vi "Write Heading Data to TDMS.vi"(8 "error in (no error)":errorcluster, 10 "Heading Data":T1, 11 "Honeywell Compass HMC6343":refnum<class "Honeywell Compass HMC6343.lvclass">) -> (0 "error out":errorcluster, 3 "Honeywell Compass HMC6343 out":refnum<class "Honeywell Compass HMC6343.lvclass">)   [LabVIEW 2019, in "Honeywell Compass HMC6343.lvclass"]
doc: "Writes Heading Data to TDMS file."
uses:
  Honeywell Compass HMC6343.lvclass
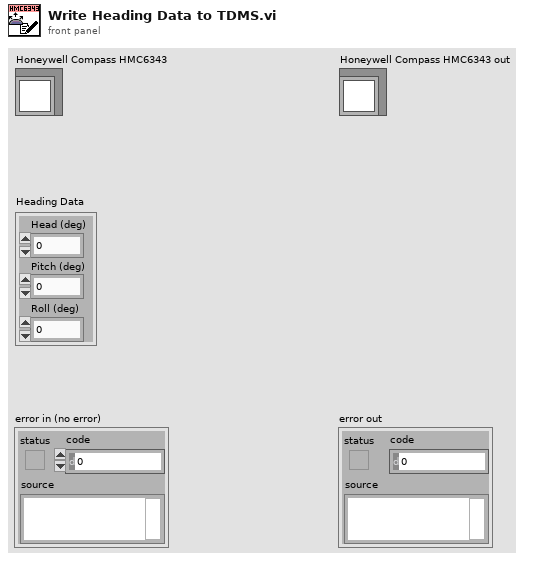
[diagram p1: front panel]
types:
  T1 = cluster{"Head (deg)":dbl, "Pitch (deg)":dbl, "Roll (deg)":dbl}
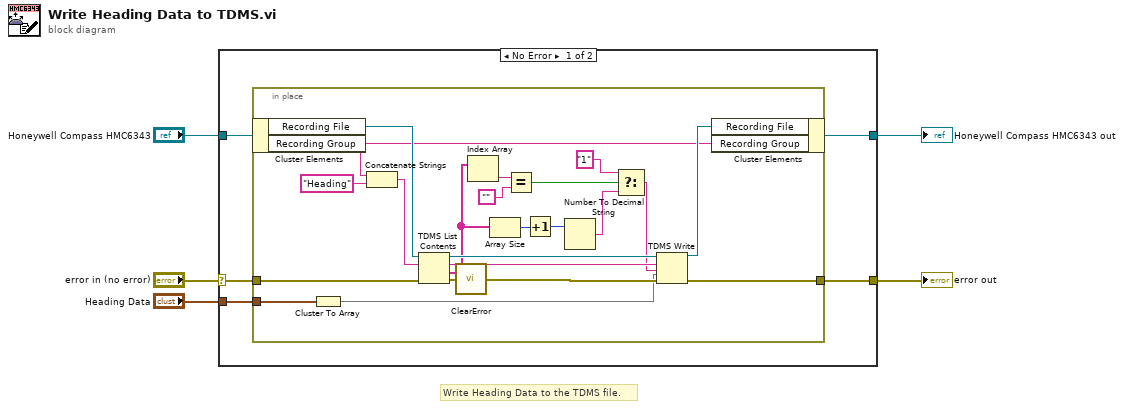
[diagram p0: block diagram]
diagram:
  # "Write Heading Data to the TDMS file."
  n1 = case shown="No Error" "error in (no error)" {
    selector: "error in (no error)" -> [w10 w33]
    tunnel: "Honeywell Compass HMC6343" -> [w9 w34]
    tunnel: [w8 w34] -> w3
    tunnel: [w7 w33] -> w2
    tunnel: "Heading Data" -> [w6 _]
    frame No Error {
      n2 = in-place "In Place Element Structure" {
        in-place-border: w10 -> [w32]
        in-place-border: [w27] -> w7
        in-place-border: w6 -> [w15]
        n3 = in-place-cluster #1(w9) -> ("Recording File"=w30:refnum<k34>, "Recording Group"=w12:string)
        n4 = Cluster To Array(cluster=w15) -> (array=w14:dbl[])
        n5 = Concatenate Strings(w12, "Heading" ("string")) -> (w16:string)
        n6 = TDMS List Contents(4:w32, 6:w16, 7:w30) -> (0:w11:errorcluster, 1:w19:string[], 2:w18:string, 3:w28:refnum<k34>)
        n7 = call <vilib>:"ClearError.vi"("error in (no error)"=w11) -> ("error out"=w31:errorcluster)
        n8 = Index Array(array=w19) -> (element=w20:string)  [unwired: 1 in]
        n9 = Array Size(array=w19) -> (size(s)=w26:i32)
        n10 = Equal?(x=w20, y="" ("Empty String Constant")) -> (x = y?=w23:bool)
        n11 = Increment(x=w26) -> (x+1=w25:i32)
        n12 = Number To Decimal String(number=w25) -> (decimal integer string=w21:string)  [unwired: 1 in]
        n13 = Select(t="1", s=w23, f=w21) -> (s? t:f=w13:string)
        n14 = TDMS Write(0:w28, 5:w18, 7:w13, 9:w14, 11:w31) -> (4:w29:refnum<k34>, 15:w27:errorcluster)  [unwired: 1 in, 2 out]
        n15 = in-place-cluster #1("Recording File"=w29, "Recording Group"=w12) -> (w8:refnum<class "Honeywell Compass HMC6343.lvclass">)
      }
    }
    frame Error {
    }
  }
  "error out" <- w2
  "Honeywell Compass HMC6343 out" <- w3
